vi "Call.vi"(7 "Actor in":refnum<class "Actor.lvclass">, 8 "Error in":errorcluster, 9 "Parent Stopped":bool, 10 "Safe Stop":bool=TRUE) -> (0 "Error out":errorcluster, 5 "Actor out":refnum<class "Actor.lvclass">)   [LabVIEW 2025, in "jettl.lvlib" / "Stop jettl Msg.lvlib" / "Stop.lvlib"]
uses:
  Stop.lvlib
  Actor/Actor.lvclass
  Init Msg.vi
  jettl.lvlib
  Stop Msg Output/Stop Msg Output.lvlib
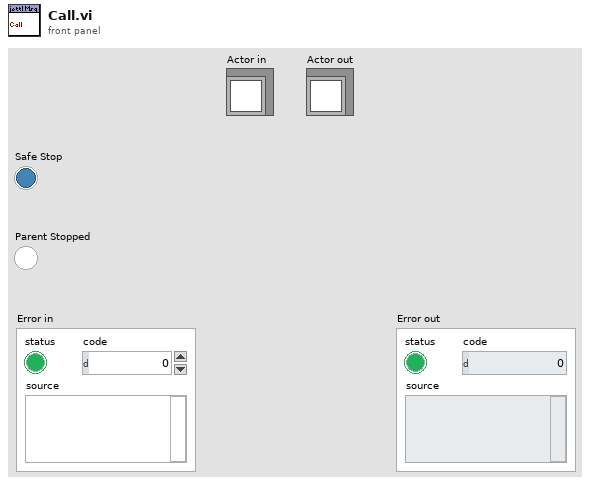
[diagram p1: front panel]
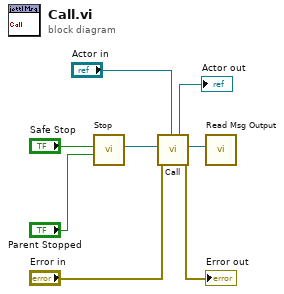
[diagram p0: block diagram]
diagram:
  n1 = call-poly "Stop.vi"("Parent Stopped"="Parent Stopped", "Safe Stop"="Safe Stop") -> ("Msg"=w3:refnum<class "Msg.lvclass">)  [unwired: 9 in]
  n2 = call "Call.vi"("Actor in"="Actor in", "Error in"="Error in", "Msg"=w3) -> ("Error out"=→"Error out":errorcluster, "Msg Output"=w4:refnum<class "Msg Output.lvclass">, "Actor out"=→"Actor out":refnum<class "Actor.lvclass">)  [unwired: 6 in]
  n3 = call "Read Msg Output.vi"("Msg Output"=w4) -> ()  [unwired: 11 in]
